vi "oa_Create Indice Interpolate.vi"(5 "reset?(F)":bool, 7 "history rev length":i32, 8 "actual steps":T1 {"step" format="%.2f"; "start" format="%.2f"}, 10 "interpolation array":dbl[](array[numeric]), 11 "reference array":dbl[](array[numeric])) -> (0 "dup actual steps":T1 {"step" format="%.2f"; "start" format="%.2f"}, 1 "interpolated values":dbl[](array[numeric]), 2 "reference values":dbl[](array[numeric]), 3 "revolution indices":dbl[](array[numeric]))   [LabVIEW 2017]
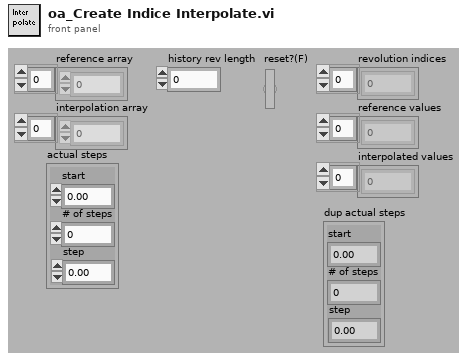
[diagram p1: front panel]
types:
  T1 = cluster{"start":dbl, "# of steps":i32, "step":dbl}
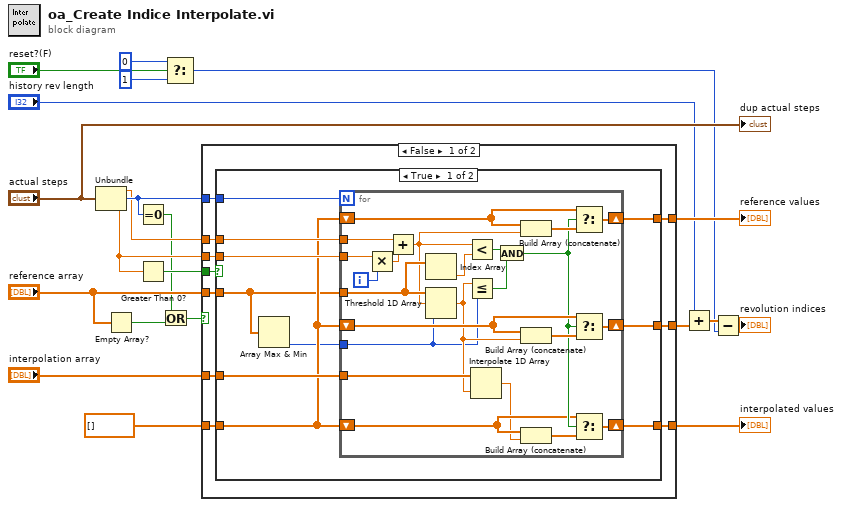
[diagram p0: block diagram]
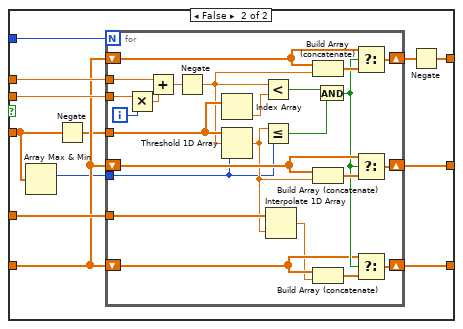
[diagram p2: hidden frame]
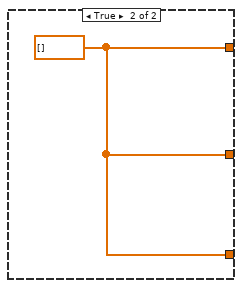
[diagram p3: hidden frame]
diagram:
  n1 = Unbundle("actual steps") -> ("start"=w19:dbl, "# of steps"=w20:i32, "step"=w7:dbl)
  n2 = Empty Array?(array="reference array") -> (empty?=w3:bool)
  n3 = Equal To 0?(x=w20) -> (x = 0?=w2:bool)
  n4 = Greater Than 0?(x=w7) -> (x > 0?=w6:bool)
  n5 = Or(x=w2, y=w3) -> (x .or. y?=w1:bool)
  n6 = Select(t=0, s="reset?(F)", f=1) -> (s? t:f=w8:i32)
  n7 = case shown="False" w1 {
    tunnel: w20 -> [w31 _]
    tunnel: "reference array" -> [w30 _]
    tunnel: w19 -> [w29 _]
    tunnel: w7 -> [w28 _]
    tunnel: [w27 w101] -> w14
    tunnel: "interpolation array" -> [w26 _]
    tunnel: [w25 w101] -> w17
    tunnel: [w24 w101] -> w16
    tunnel: w6 -> [w23 _]
    tunnel: dbl[] [] -> [w22 _]
    frame False {
      n8 = case shown="True" w23 {
        tunnel: w31 -> [w41 w76]
        tunnel: w30 -> [w33 w66]
        tunnel: w29 -> [w40 w75]
        tunnel: w28 -> [w39 w74]
        tunnel: [w36 w67] -> w27
        tunnel: w26 -> [w38 w73]
        tunnel: [w35 w71] -> w25
        tunnel: [w37 w68] -> w24
        tunnel: w22 -> [w34 w70]
        frame True {
          n9 = Array Max & Min(array=w33) -> (min index (indices)=w32:i32)  [unwired: 3 out]
          n10 = for {
            N: w41 -> [_]
            tunnel: w33 -> [w58]
            tunnel: w40 -> [w64]
            tunnel: w39 -> [w63]
            tunnel: w38 -> [w60]
            shift-right: [w55] -> w37
            shift-left: w34 -> [w53]
            shift-right: [w50] -> w36
            shift-left: w34 -> [w49]
            shift-right: [w46] -> w35
            shift-left: w34 -> [w45]
            tunnel: w32 -> [w42]
            i -> [w62]
            n11 = Multiply(x=w63, y=w62) -> (x*y=w61:dbl)
            n12 = Add(x=w64, y=w61) -> (x+y=w54:dbl)
            n13 = Index Array(array=w58) -> (element=w59:dbl)  [unwired: 1 in]
            n14 = Threshold 1D Array(1:w42, 2:w54, 3:w58) -> (0:w43:dbl)
            n15 = Less?(x=w54, y=w59) -> (x < y?=w57:bool)
            n16 = Less Or Equal?(x=w43, y=w42) -> (x <= y?=w56:bool)
            n17 = Interpolate 1D Array(1:w43, 2:w60) -> (0:w44:dbl)
            n18 = And(x=w57, y=w56) -> (x .and. y?=w47:bool)
            n19 = Build Array (concatenate)(w53, w54) -> (w52:dbl[])
            n20 = Build Array (concatenate)(w49, w43) -> (w51:dbl[])
            n21 = Build Array (concatenate)(w45, w44) -> (w48:dbl[])
            n22 = Select(t=w53, s=w47, f=w52) -> (s? t:f=w55:dbl[])
            n23 = Select(t=w49, s=w47, f=w51) -> (s? t:f=w50:dbl[])
            n24 = Select(t=w45, s=w47, f=w48) -> (s? t:f=w46:dbl[])
          }
        }
        frame False {
          n25 = Array Max & Min(array=w66) -> (max index (indices)=w65:i32)  [unwired: 3 out]
          n26 = Negate(x=w66) -> (-x=w69:dbl[])
          n27 = for {
            N: w76 -> [_]
            tunnel: w69 -> [w94]
            tunnel: w75 -> [w100]
            tunnel: w74 -> [w99]
            tunnel: w73 -> [w96]
            shift-right: [w92] -> w72
            shift-left: w70 -> [w90]
            shift-right: [w87] -> w67
            shift-left: w70 -> [w86]
            shift-right: [w82] -> w71
            shift-left: w70 -> [w81]
            tunnel: w65 -> [w77]
            i -> [w98]
            n28 = Multiply(x=w99, y=w98) -> (x*y=w97:dbl)
            n29 = Add(x=w100, y=w97) -> (x+y=w91:dbl)
            n30 = Negate(x=w91) -> (-x=w79:dbl)
            n31 = Index Array(array=w94) -> (element=w95:dbl)  [unwired: 1 in]
            n32 = Threshold 1D Array(1:w77, 2:w79, 3:w94) -> (0:w85:dbl)
            n33 = Less?(x=w79, y=w95) -> (x < y?=w93:bool)
            n34 = Less Or Equal?(x=w85, y=w77) -> (x <= y?=w78:bool)
            n35 = Interpolate 1D Array(1:w85, 2:w96) -> (0:w80:dbl)
            n36 = Build Array (concatenate)(w90, w79) -> (w89:dbl[])
            n37 = Build Array (concatenate)(w86, w85) -> (w88:dbl[])
            n38 = Build Array (concatenate)(w81, w80) -> (w84:dbl[])
            n39 = And(x=w93, y=w78) -> (x .and. y?=w83:bool)
            n40 = Select(t=w90, s=w83, f=w89) -> (s? t:f=w92:dbl[])
            n41 = Select(t=w86, s=w83, f=w88) -> (s? t:f=w87:dbl[])
            n42 = Select(t=w81, s=w83, f=w84) -> (s? t:f=w82:dbl[])
          }
          n43 = Negate(x=w72) -> (-x=w68:dbl[])
        }
      }
    }
    frame True {
      w101 = dbl[] []
    }
  }
  "reference values" <- w16
  "interpolated values" <- w17
  n44 = Add(x="history rev length", y=w14) -> (x+y=w9:dbl[])
  n45 = Subtract(x=w9, y=w8) -> (x-y=→"revolution indices":dbl[])
  "dup actual steps" <- "actual steps"
